vi "ADIS16470 Scale Data Register.vi"(5 "DeltaTimeStamp":dbl, 10 "Data In":u16[](array[numeric])) -> (1 "Temp_DegC":dbl, 2 "DiagStat":u16, 3 "Scaled Data Out":dbl[](array[numeric]))   [LabVIEW 2019]
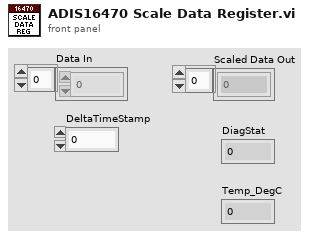
[diagram p1: front panel]
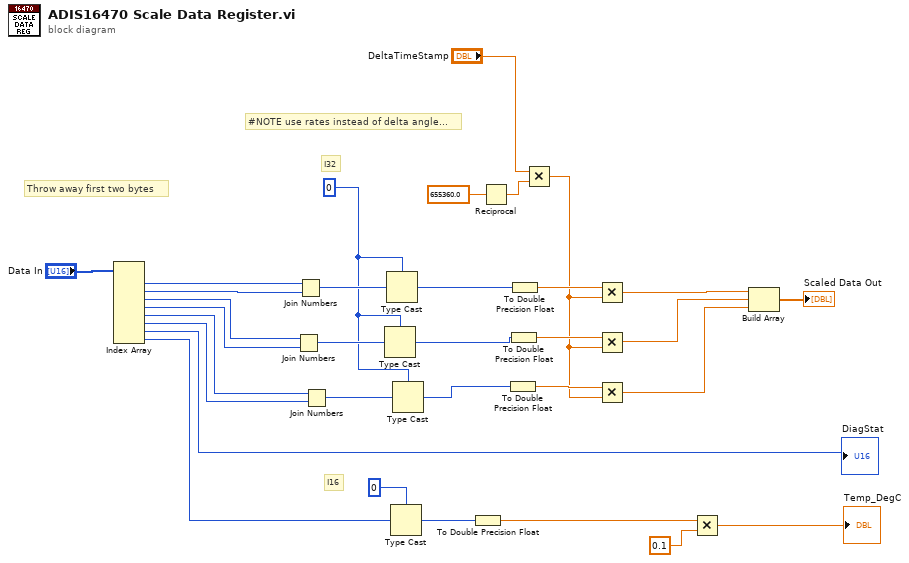
[diagram p0: block diagram]
diagram:
  w11 = 0
  # "#NOTE use rates instead of delta angle..."
  # "I16"
  # "I32"
  # "Throw away first two bytes"
  n1 = Index Array(array="Data In") -> (element #1=w28:u16, element #2=w27:u16, element #3=w26:u16, element #4=w25:u16, element #5=w24:u16, element #6=w23:u16, element #7=→"DiagStat":u16, element #8=w20:u16)  [unwired: 8 in]
  n2 = Join Numbers(hi=w26, lo=w25) -> ((hi.lo)=w30:u32)
  n3 = Join Numbers(hi=w28, lo=w27) -> ((hi.lo)=w31:u32)
  n4 = Join Numbers(hi=w24, lo=w23) -> ((hi.lo)=w29:u32)
  n5 = Type Cast(type=w11, x=w30) -> (*(type *) &x=w9:i32)
  n6 = Type Cast(type=w11, x=w31) -> (*(type *) &x=w10:i32)
  n7 = Type Cast(type=i16 0, x=w20) -> (*(type *) &x=w19:i16)
  n8 = Type Cast(type=w11, x=w29) -> (*(type *) &x=w8:i32)
  n9 = To Double Precision Float(number=w19) -> (double precision float=w14:dbl)
  n10 = Reciprocal(x=655360.0) -> (1/x=w7:dbl)
  n11 = To Double Precision Float(number=w8) -> (double precision float=w16:dbl)
  n12 = To Double Precision Float(number=w9) -> (double precision float=w17:dbl)
  n13 = To Double Precision Float(number=w10) -> (double precision float=w18:dbl)
  n14 = Multiply(x="DeltaTimeStamp", y=w7) -> (x*y=w5:dbl)
  n15 = Multiply(x=w18, y=w5) -> (x*y=w4:dbl)
  n16 = Multiply(x=w17, y=w5) -> (x*y=w2:dbl)
  n17 = Multiply(x=w16, y=w5) -> (x*y=w1:dbl)
  n18 = Multiply(x=w14, y=0.1) -> (x*y=→"Temp_DegC":dbl)
  n19 = Build Array(w4, w2, w1) -> (→"Scaled Data Out":dbl[])
